vi "Insert Stop Message.vi"(8 "error in (no error)":errorcluster, 11 "BehaviorData in":refnum<class "BehaviorData.lvclass">) -> (0 "error out":errorcluster, 3 "BehaviorData out":refnum<class "BehaviorData.lvclass">)   [LabVIEW 2010, in "BehaviorData.lvclass"]
uses:
  BehaviorData.lvclass
  Database/BehPrimary.ctl
  AcquistionObject/AcquistionObject.lvclass
  <vilib>/addons/database/NI_Database_API.lvlib
panel:
  out "resulting string":string
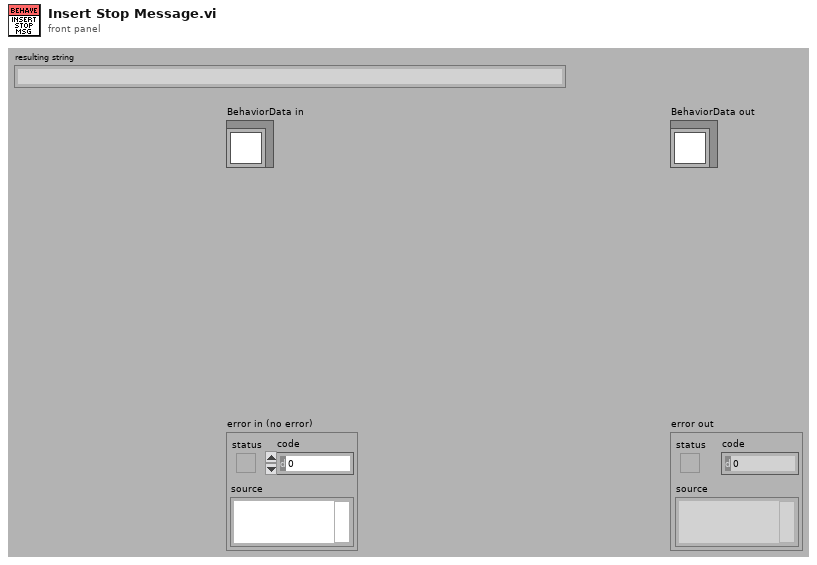
[diagram p1: front panel]
types:
  T1 = typedef "BehPrimary.ctl" = cluster{"setup":u8, "session_start_time":dbl, "stim_start_time":dbl, "beh_start_time":dbl}
  T2 = typedef "NI_Database_API.lvlib/Conn ObjectReference.ctl" = refnum<k1>
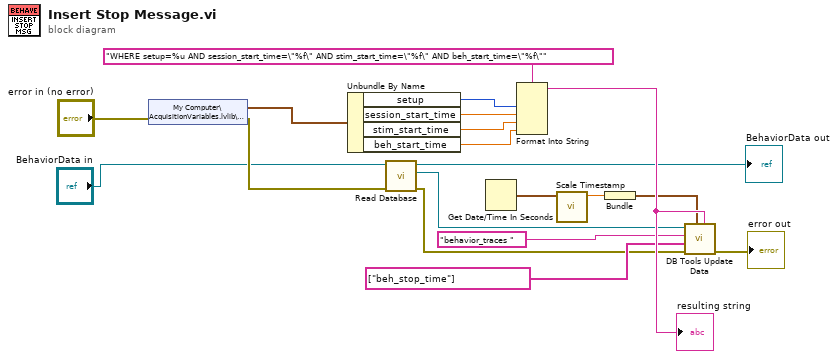
[diagram p0: block diagram]
diagram:
  n1 = shared-variable "My Computer\\AcquisitionVariables.lvlib\\BehaviorPK"(error in="error in (no error)") -> (w18:T1, error out=w8:errorcluster)
  n2 = Unbundle By Name(w18) -> ("setup"=w16:u8, "session_start_time"=w15:dbl, "stim_start_time"=w6:dbl, "beh_start_time"=w1:dbl)
  n3 = call-dynamic "Read Database.vi"("error in (no error)"=w8, "AcquistionObject in"="BehaviorData in") -> ("error out"=w7:errorcluster, "reference"=w10:T2, "AcquistionObject out"=→"BehaviorData out":refnum<class "BehaviorData.lvclass">)  [unwired: 7 in]
  n4 = Get Date/Time In Seconds() -> (seconds since 1Jan1904=w19:timestamp)
  n5 = Format Into String(format string="WHERE setup=%u AND session_start_time=\"%f\" AND stim_start_time=\"%f\" AND beh_start_time=\"%f\"", w16, w15, w6, w1) -> (resulting string=w14:string)  [unwired: 2 in, 1 out]
  "resulting string" <- w14
  n6 = call "Scale Timestamp.vi"("Time Stamp"=w19) -> ("Scaled timestamp"=w11:dbl)  [unwired: 10 in]
  n7 = Bundle("Scaled timestamp"=w11) -> (w12:cluster{"Scaled timestamp":dbl})  [unwired: 1 in]
  n8 = call <vilib>:"DB Tools Update Data.vi"("condition"=w14, "data"=w12, "error in (no error)"=w7, "columns"=string[] ["beh_stop_time"], "table"="behavior_traces ", "connection reference"=w10) -> ("error out"=→"error out":errorcluster)  [unwired: 4 in, 1 out]
